vi "Normal.vi"(11 "Triangle":T2={"Vertex 1"={"Position"={"x"=0.0, "y"=0.0, "z"=0.0}, "UV"={"u"=0.0, "v"=0.0}, "Colour"=12517256}, "Vertex 2"={"Position"={"x"=0.0, "y"=0.0, "z"=0.0}, "UV"={"u"=0.0, "v"=0.0}, "Colour"=12517256}, "Vertex 3"={"Position"={"x"=0.0, "y"=0.0, "z"=0.0}, "UV"={"u"=0.0, "v"=0.0}, "Colour"=12517256}, "Alpha"=0.0, "Alpha Blending Enabled"=FALSE, "Colour"=0, "Material"={"Diffuse Colour"=0, "Texture"={"Pixels"=refnum, "Size"={"Width"=0, "Height"=0}}}} {"Vertex 3"."UV"."v" min=0 max=1 step=0.1; "Vertex 3"."UV"."u" min=0 max=1 step=0.1; "Vertex 2"."UV"."v" min=0 max=1 step=0.1; "Vertex 2"."UV"."u" min=0 max=1 step=0.1; "Vertex 1"."UV"."v" min=0 max=1 step=0.1; "Vertex 1"."UV"."u" min=0 max=1 step=0.1}) -> (3 "Normal":T1)   [LabVIEW 2020, in "3D (FPGA).lvlib"]
uses:
  3D (FPGA).lvlib
  Vector 3D.ctl
  Raster/UV.ctl
  Raster/Raster (FPGA).lvlib
  Vertex.ctl
  Triangle.ctl
  Raster/Rectangle Dimensions.ctl
  Raster/Texture.ctl
  Material.ctl
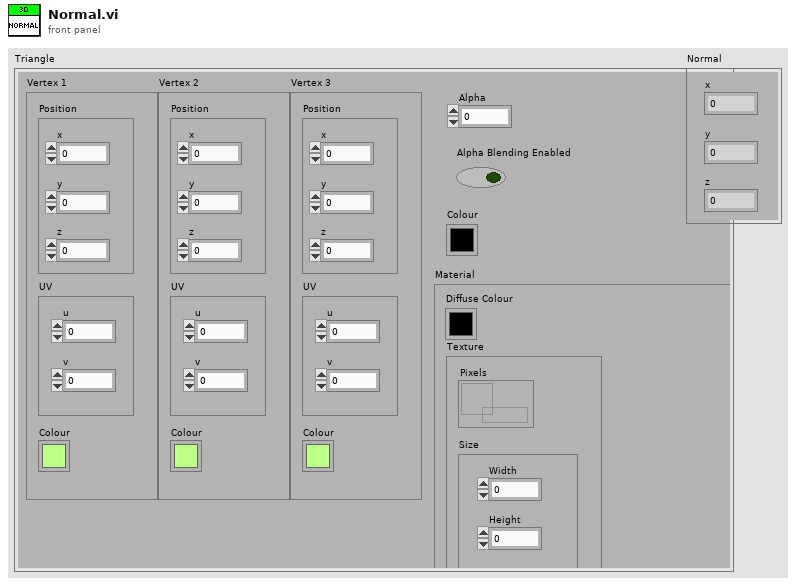
[diagram p1: front panel]
types:
  T1 = typedef "3D (FPGA).lvlib/Vector 3D.ctl" = cluster{"x":sgl, "y":sgl, "z":sgl}
  T2 = typedef "3D (FPGA).lvlib/Triangle.ctl" = cluster{"Vertex 1":T3, "Vertex 2":T3, "Vertex 3":T3, "Alpha":dbl, "Alpha Blending Enabled":bool, "Colour":u32, "Material":T5}
  T3 = typedef "3D (FPGA).lvlib/Vertex.ctl" = cluster{"Position":T1, "UV":T4, "Colour":u32}
  T4 = typedef "Raster (FPGA).lvlib/UV.ctl" = cluster{"u":sgl, "v":sgl}
  T5 = typedef "3D (FPGA).lvlib/Material.ctl" = cluster{"Diffuse Colour":u32, "Texture":T6}
  T6 = typedef "Raster (FPGA).lvlib/Texture.ctl" = cluster{"Pixels":refnum<data-value>, "Size":T7}
  T7 = typedef "Raster (FPGA).lvlib/Rectangle Dimensions.ctl" = cluster{"Width":u32, "Height":u32}
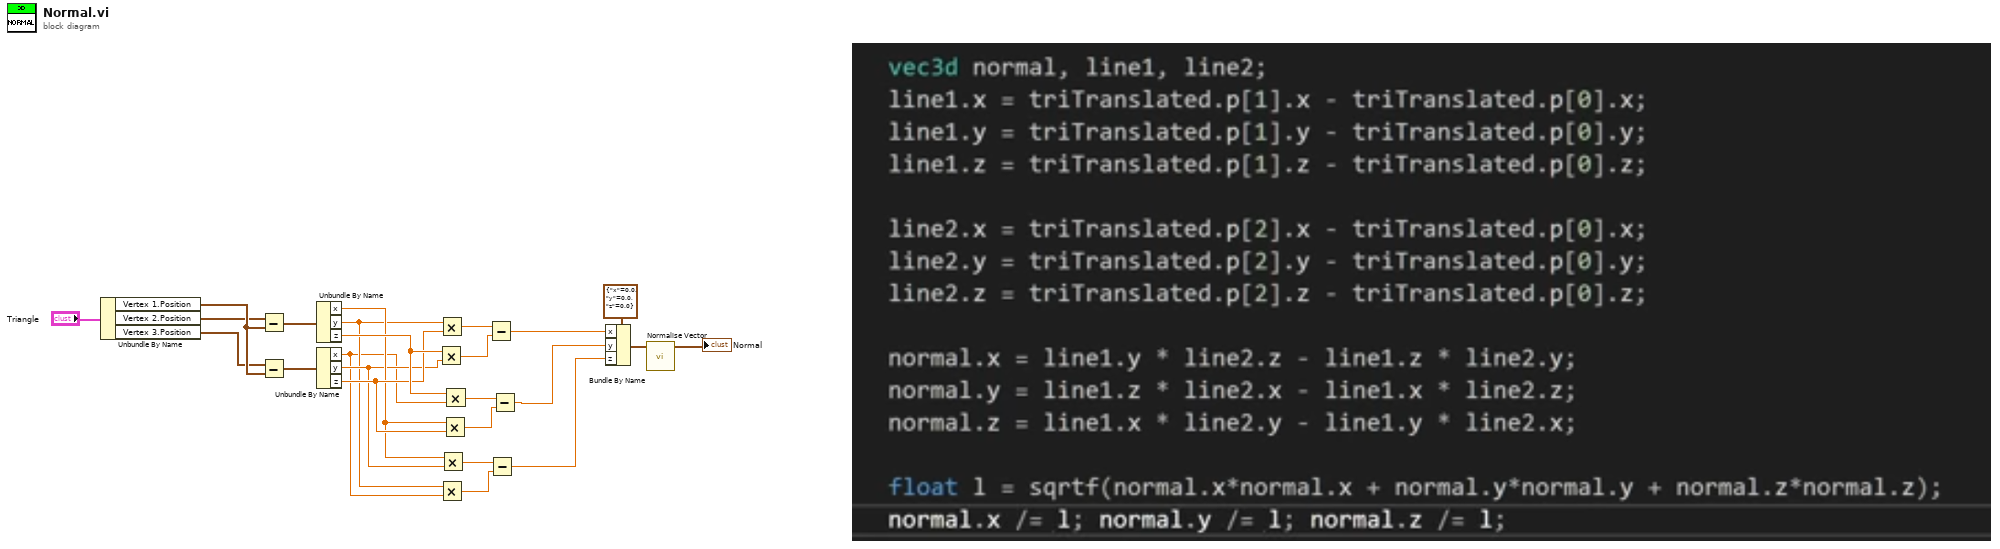
[diagram p0: block diagram]
diagram:
  n1 = Unbundle By Name("Triangle") -> ("Vertex 1.Position"=w3:T1, "Vertex 2.Position"=w2:T1, "Vertex 3.Position"=w1:T1)
  n2 = Subtract(x=w2, y=w3) -> (x-y=w22:T1)
  n3 = Subtract(x=w1, y=w3) -> (x-y=w21:T1)
  n4 = Unbundle By Name(w22) -> ("x"=w9:sgl, "y"=w7:sgl, "z"=w11:sgl)
  n5 = Unbundle By Name(w21) -> ("x"=w6:sgl, "y"=w8:sgl, "z"=w10:sgl)
  n6 = Multiply(x=w11, y=w8) -> (x*y=w19:sgl)
  n7 = Multiply(x=w7, y=w10) -> (x*y=w20:sgl)
  n8 = Multiply(x=w7, y=w6) -> (x*y=w14:sgl)
  n9 = Multiply(x=w9, y=w8) -> (x*y=w15:sgl)
  n10 = Multiply(x=w9, y=w10) -> (x*y=w17:sgl)
  n11 = Multiply(x=w11, y=w6) -> (x*y=w16:sgl)
  n12 = Subtract(x=w20, y=w19) -> (x-y=w18:sgl)
  n13 = Subtract(x=w15, y=w14) -> (x-y=w12:sgl)
  n14 = Subtract(x=w16, y=w17) -> (x-y=w13:sgl)
  n15 = Bundle By Name(cluster=T1 {"x"=0.0, "y"=0.0, "z"=0.0} ("Normal"), "x"=w18, "y"=w13, "z"=w12) -> (w5:T1)
  n16 = call "Normalise Vector.vi"("Vector 3D"=w5) -> ("Vector 3D Normalised"=→"Normal":T1)  [unwired: 10 in]
